vi "Probe 3 bits DIO26-28 D3-5.vi"(9 "U8":u8) -> ()   [LabVIEW 2017]
uses:
  <vilib>/rvi/eio/common/nirviEmuTemplateMethod_errors.vi
  <vilib>/eio/EIONode/EIONode.xnode
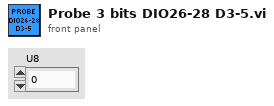
[diagram p1: front panel]
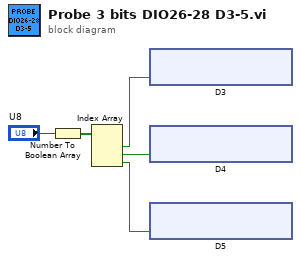
[diagram p0: block diagram]
diagram:
  n1 = Number To Boolean Array(number="U8") -> (Boolean array=w3:bool[])
  n2 = Index Array(array=w3) -> (element #1=w2:bool, element #2=w1:bool, element #3=w4:bool)  [unwired: 3 in]
  n3 = xnode "D3"("Connector0/DIO28"=w2) -> ()  [unwired: 1 in, 1 out]
  n4 = xnode "D4"("Connector0/DIO27"=w1) -> ()  [unwired: 1 in, 1 out]
  n5 = xnode "D5"("Connector0/DIO26"=w4) -> ()  [unwired: 1 in, 1 out]
